vi "Serial Number to Port.vi"(0 "Port In":string) -> (1 "Port Out":string, 2 "error out":errorcluster)   [LabVIEW 2021]
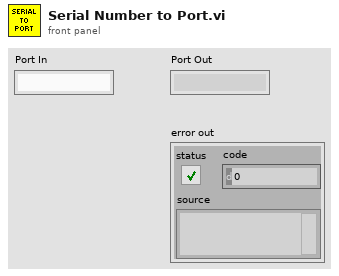
[diagram p1: front panel]
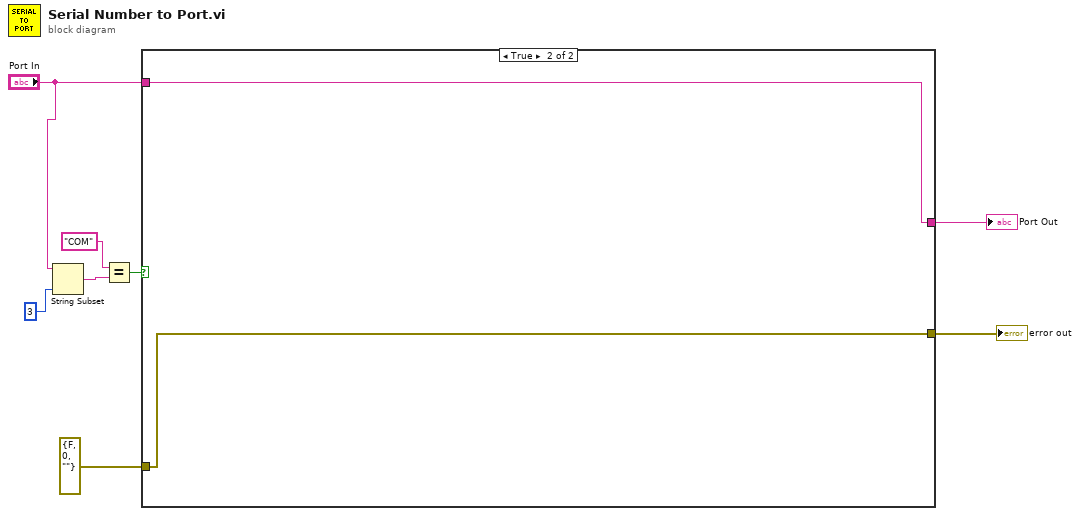
[diagram p0: block diagram]
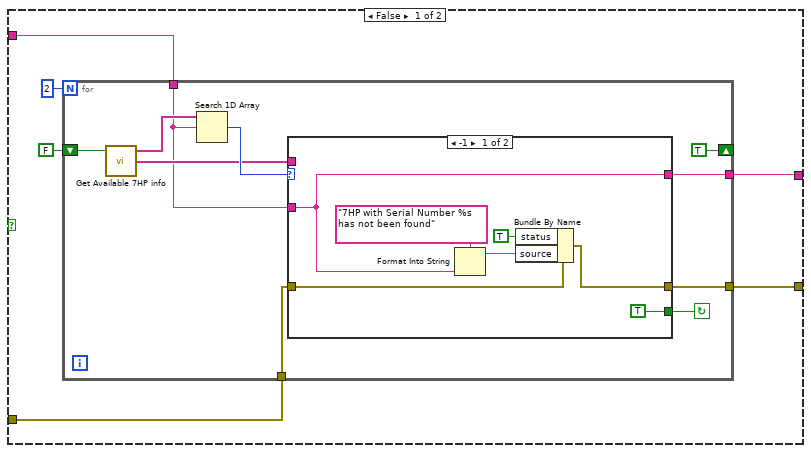
[diagram p2: hidden frame]
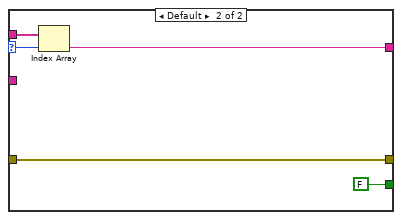
[diagram p3: hidden frame]
diagram:
  n1 = String Subset(string="Port In", length (rest)=3 ("length (rest)")) -> (substring=w4:string)  [unwired: 1 in]
  n2 = Equal?(x="COM", y=w4) -> (x = y?=w2:bool)
  n3 = case shown="True" w2 {
    tunnel: [w14 w38] -> w8
    tunnel: [w13 w37] -> w7
    tunnel: "Port In" -> [w10 w38]
    tunnel: errorcluster {"status"=FALSE, "code"=0, "source"=""} ("error out") -> [w9 w37]
    frame False {
      n4 = for {
        N: 2 -> [_]
        tunnel: [w24] -> w14
        tunnel: [w20] -> w13
        shift-right: [TRUE] -> _
        shift-left: FALSE -> [w17]
        tunnel: w10 -> [w16]
        tunnel: w9 -> [w15]
        stop <- w19 continue-if-true
        n5 = call "Get Available 7HP info.vi"("Force Another Read"=w17) -> ("7HP Port names"=w21:string[], "7HP Serial numbers"=w22:string[])  [unwired: 2 in, 1 out]
        n6 = Search 1D Array(1D array=w22, element=w16) -> (index of element=w23:i32)  [unwired: 1 in]
        n7 = case shown="-1" w23 {
          selector: w23 -> [_ w35]
          tunnel: [w29 w36] -> w24
          tunnel: w16 -> [w29 _]
          tunnel: w21 -> [_ w34]
          tunnel: [w31 w33] -> w20
          tunnel: w15 -> [w30 w33]
          tunnel: [TRUE FALSE] -> w19
          frame -1 {
            n8 = Format Into String(format string="7HP with Serial Number %s has not been found", w29) -> (resulting string=w26:string)  [unwired: 2 in, 1 out]
            n9 = Bundle By Name(cluster=w30, "status"=TRUE, "source"=w26) -> (w31:errorcluster)
          }
          frame Default {
            n10 = Index Array(array=w34, index=w35) -> (element=w36:string)
          }
        }
      }
    }
    frame True {
    }
  }
  "Port Out" <- w8
  "error out" <- w7
